vi "concatenate arrays.vi"(10 "Array 2":dbl[](array[numeric]), 11 "Array 1":dbl[](array[numeric])) -> (0 "output array 2":dbl[](array[numeric]))   [LabVIEW 2010]
panel:
  out "output array":dbl[](array[numeric])
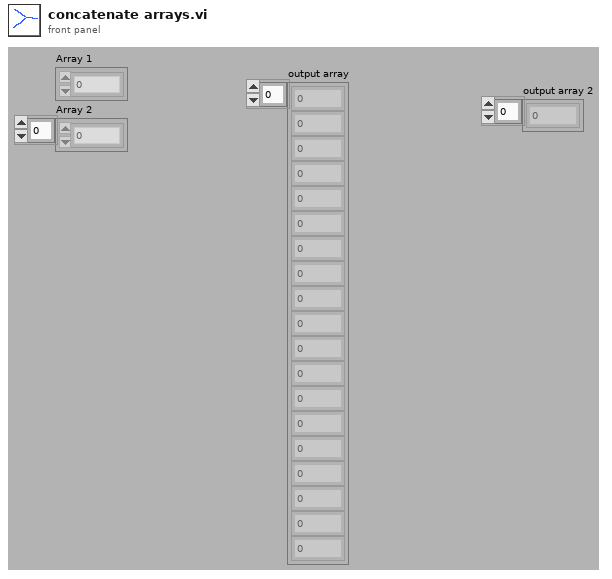
[diagram p1: front panel]
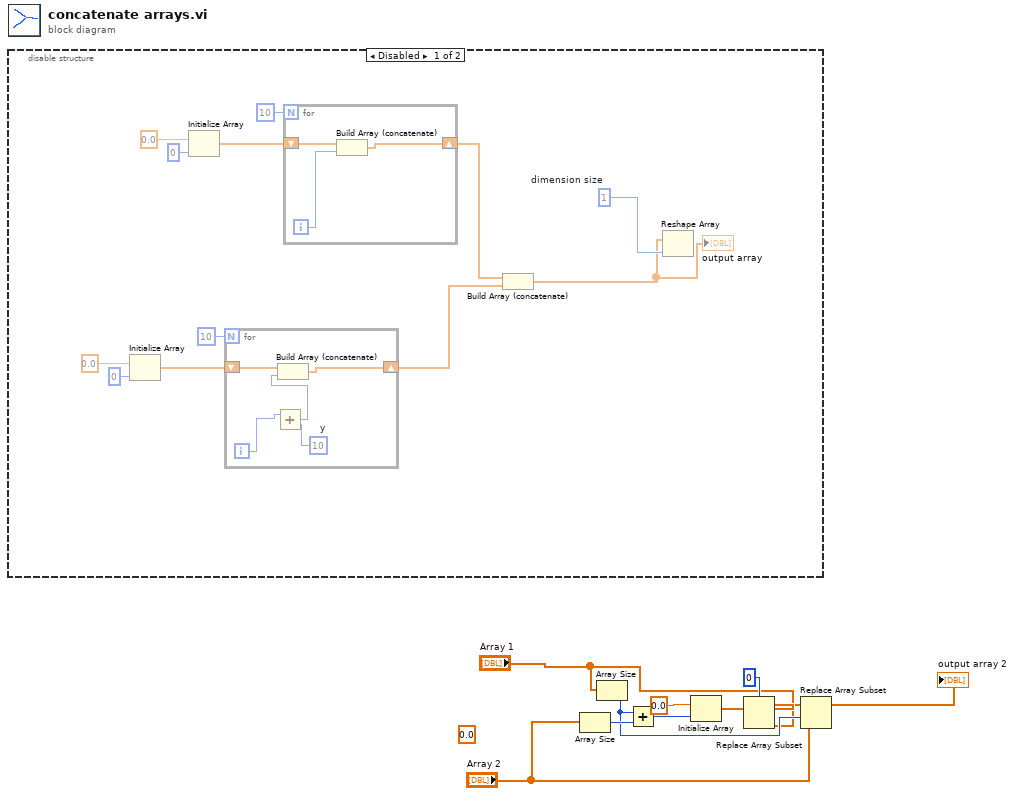
[diagram p0: block diagram]
diagram:
  (unwired) 0.0 ("dimension size")
  n1 = disable-structure shown="Disabled" {
    frame Disabled {
      w14 = 1  # dimension size
      n2 = Initialize Array(0.0 ("dimension size"), 0 ("dimension size")) -> (w16:dbl[])
      n3 = Initialize Array(0.0 ("dimension size"), 0 ("dimension size")) -> (w20:dbl[])
      n4 = for {
        N: 10 -> [_]
        shift-right: [w26] -> w13
        shift-left: w16 -> [w27]
        i -> [w25]
        w24 = 10  # y
        n5 = Add(x=w25, y=w24) -> (x+y=w23:i32)
        n6 = Build Array (concatenate)(w27, w23) -> (w26:dbl[])
      }
      n7 = for {
        N: 10 -> [_]
        shift-right: [w28] -> w11
        shift-left: w20 -> [w30]
        i -> [w29]
        n8 = Build Array (concatenate)(w30, w29) -> (w28:dbl[])
      }
      n9 = Build Array (concatenate)(w11, w13) -> (w12:dbl[])
      "output array" <- w12
      n10 = Reshape Array(w12, w14) -> ()  [unwired: 1 out]
    }
    frame Enabled {
    }
  }
  n11 = Array Size(array="Array 2") -> (size(s)=w9:i32)
  n12 = Array Size(array="Array 1") -> (size(s)=w4:i32)
  n13 = Add(x=w4, y=w9) -> (x+y=w8:i32)
  n14 = Initialize Array(0.0 ("dimension size"), w8) -> (w7:dbl[])
  n15 = Replace Array Subset(array=w7, new element="Array 1", index=0 ("dimension size")) -> (w5:dbl[])
  n16 = Replace Array Subset(array=w5, new element="Array 2", index=w4) -> (→"output array 2":dbl[])
